vi "Register User Events.vi"(8 "error in (no error)":errorcluster, 11 "UI in":refnum<class "UI.lvclass">) -> (0 "error out":errorcluster)   [LabVIEW 2015, in "UI.lvlib" / "UI.lvclass"]
uses:
  UI.lvclass
  <vilib>/ActorFramework/Message Enqueuer/Message Enqueuer.lvclass
  <vilib>/vision/Image Controls.llb/IMAQ Image.ctl
panel:
  out "Event Reg Refnum":refnum<event-registration>
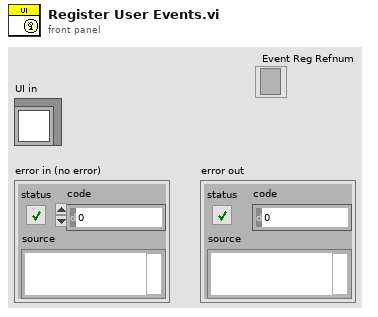
[diagram p1: front panel]
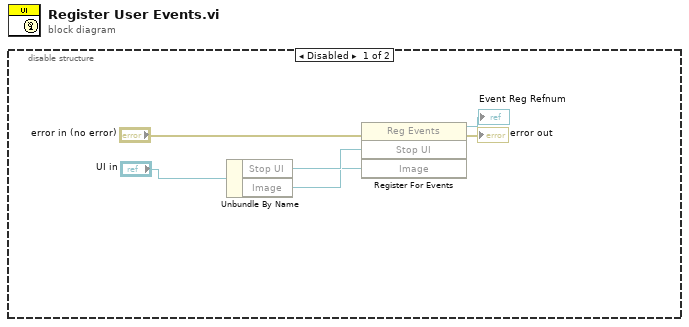
[diagram p0: block diagram]
diagram:
  n1 = disable-structure shown="Disabled" {
    frame Disabled {
      n2 = Unbundle By Name("UI in") -> ("Stop UI"=w3:refnum<user-event>, "Image"=w2:refnum<user-event>)
      n3 = register-events(error in="error in (no error)", w3, w2) -> (reference out=→"Event Reg Refnum":refnum<event-registration>, error out=→"error out":errorcluster)  [unwired: 1 in]
    }
    frame Enabled {
    }
  }
